vi "Update_Enum (SubVI).vi"(8 "error in":errorcluster, 11 "AppContext in":T1={"VIRefToProcessTemplate"=refnum, "VIRefToThisVI"=refnum, "ProcessesList"=[], "VIRefToEnumProcess"=refnum, "VIRefTogetProcessViPath"=refnum, "ProcessManagement"={"EnumProcessState"=enum."Create process", "ProcessName"="", "PathToProcess"=path ""}, "VIRefToSetup"=refnum, "VIRefToStartProcess"=refnum, "ProcessConfig"={"File Path Control"=path "", "Timeout"=0.0, "viInitString"="", "State"=enum."Closed"}}) -> (0 "error out":errorcluster, 3 "AppContext out":T1={"VIRefToProcessTemplate"=refnum, "VIRefToThisVI"=refnum, "ProcessesList"=[], "VIRefToEnumProcess"=refnum, "VIRefTogetProcessViPath"=refnum, "ProcessManagement"={"EnumProcessState"=enum."Create process", "ProcessName"="", "PathToProcess"=path ""}, "VIRefToSetup"=refnum, "VIRefToStartProcess"=refnum, "ProcessConfig"={"File Path Control"=path "", "Timeout"=0.0, "viInitString"="", "State"=enum."Closed"}})   [LabVIEW 2013]
uses:
  Ctl/AppContext.ctl
  Ctl/EnumProcessState.ctl
  050 - CONFIG/20 - ExternalProcesses/paramsExternalProcesses.ctl
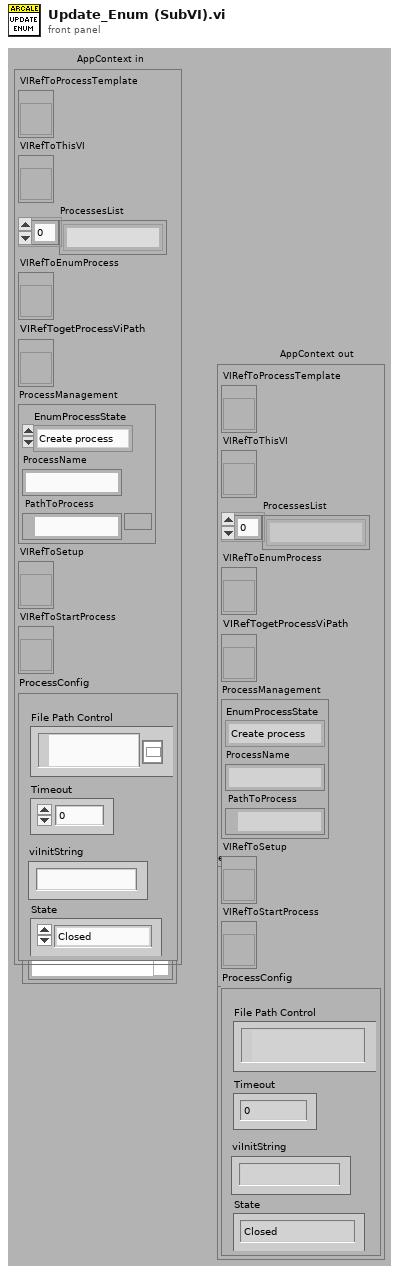
[diagram p1: front panel]
types:
  T1 = typedef "AppContext.ctl" = cluster{"VIRefToProcessTemplate":refnum<vi>, "VIRefToThisVI":refnum<vi>, "ProcessesList":string[], "VIRefToEnumProcess":refnum<vi>, "VIRefTogetProcessViPath":refnum<vi>, "ProcessManagement":cluster{"EnumProcessState":T2, "ProcessName":string, "PathToProcess":path}, "VIRefToSetup":refnum<vi>, "VIRefToStartProcess":refnum<vi>, "ProcessConfig":T3}
  T2 = typedef "EnumProcessState.ctl" = enum16{"Create process", "Delete process"}
  T3 = typedef "paramsExternalProcesses.ctl" = cluster{"File Path Control":path, "Timeout":dbl, "viInitString":string, "State":enum32{"Invalid", "Standard", "Closed", "Hidden", "Minimized", "Maximized"}}
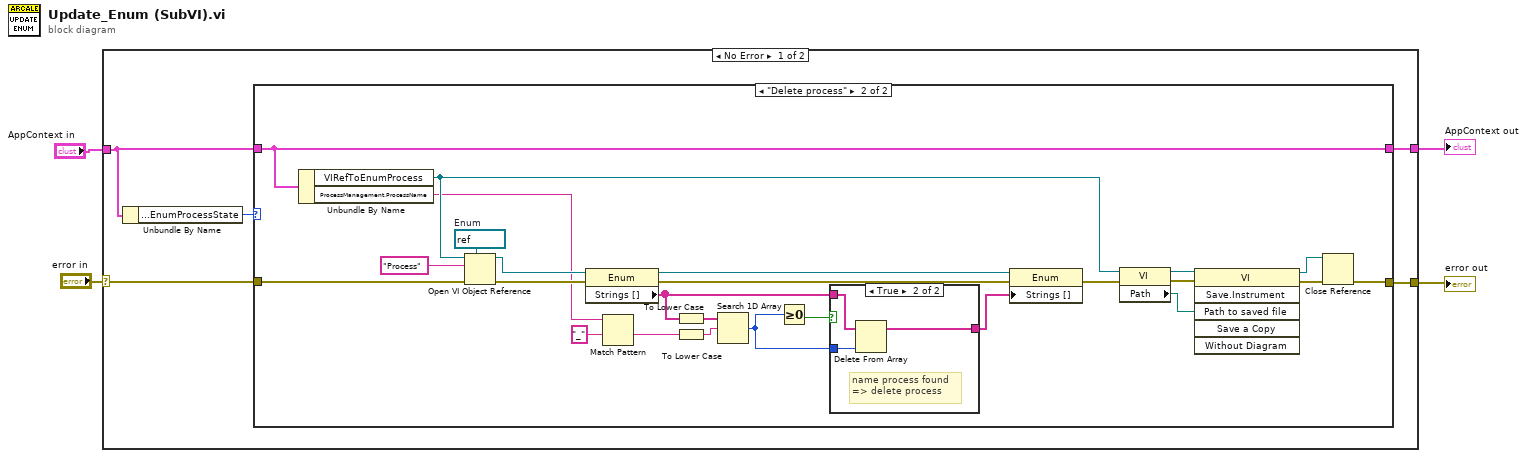
[diagram p0: block diagram]
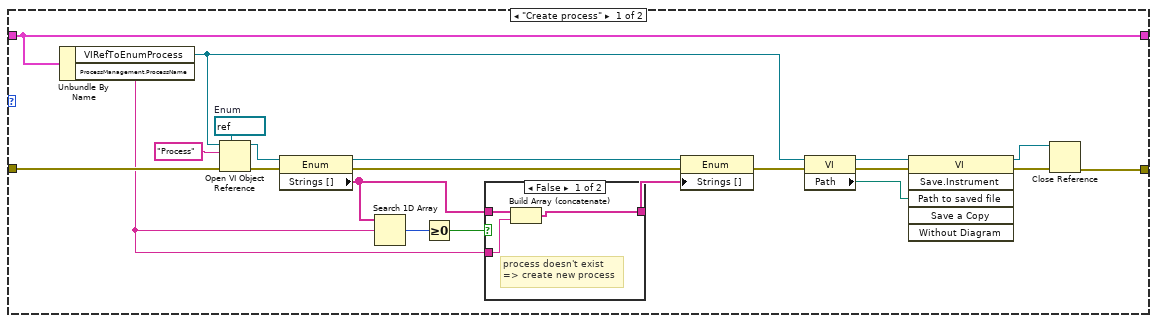
[diagram p2: hidden frame]
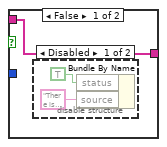
[diagram p4: hidden frame]
diagram:
  n1 = case shown="No Error" "error in" {
    selector: "error in" -> [w5 w66]
    tunnel: [w9 w66] -> w4
    tunnel: "AppContext in" -> [w7 w67]
    tunnel: [w6 w67] -> w2
    frame No Error {
      n2 = Unbundle By Name(w7) -> ("ProcessManagement.EnumProcessState"=w8:T2)
      n3 = case shown="\"Delete process\"" w8 {
        tunnel: w7 -> [w22 w51]
        tunnel: w5 -> [w29 w52]
        tunnel: [w20 w36] -> w9
        tunnel: [w22 w51] -> w6
        frame "Create process" {
          w26 = refnum<vi> refnum  # Enum
          n4 = Unbundle By Name(w22) -> ("VIRefToEnumProcess"=w24:refnum<vi>, "ProcessManagement.ProcessName"=w15:string)
          n5 = Open VI Object Reference(7:w26, 8:w29, 10:"Process" ("name/order"), 11:w24) -> (0:w19:errorcluster, 3:w25:refnum<vi>)
          n6 = property class="Enum"(reference=w25, error in=w19) -> (reference out=w28:refnum<vi>, error out=w27:errorcluster, "Strings []"=w16:string[])
          n7 = Search 1D Array(1D array=w16, element=w15) -> (index of element=w18:i32)  [unwired: 1 in]
          n8 = Greater Or Equal To 0?(x=w18) -> (x >= 0?=w17:bool)
          n9 = case shown="False" w17 {
            tunnel: w16 -> [w33 w34]
            tunnel: w15 -> [w32 _]
            tunnel: [w31 w34] -> w14
            frame False {
              # "process doesn't exist\n=> create new process"
              n10 = Build Array (concatenate)(w33, w32) -> (w31:string[])
            }
            frame True {
            }
          }
          n11 = property class="Enum"(reference=w28, error in=w27, "Strings []"=w14) -> (error out=w12:errorcluster)  [unwired: 1 out]
          n12 = property class="VI"(reference=w24, error in=w12) -> (reference out=w13:refnum<vi>, error out=w11:errorcluster, "Path"=w23:path)
          n13 = invoke class="VI" method="Save.Instrument"(reference=w13, error in=w11, "Path to saved file"=w23) -> (reference out=w21:refnum<vi>, error out=w10:errorcluster)  [unwired: 3 in, 4 out]
          n14 = Close Reference(reference=w21, error in (no error)=w10) -> (error out=w20:errorcluster)
        }
        frame "Delete process" {
          w56 = refnum<vi> refnum  # Enum
          n15 = Unbundle By Name(w51) -> ("VIRefToEnumProcess"=w54:refnum<vi>, "ProcessManagement.ProcessName"=w46:string)
          n16 = Open VI Object Reference(7:w56, 8:w52, 10:"Process" ("name/order"), 11:w54) -> (0:w47:errorcluster, 3:w55:refnum<vi>)
          n17 = property class="Enum"(reference=w55, error in=w47) -> (reference out=w58:refnum<vi>, error out=w57:errorcluster, "Strings []"=w45:string[])
          n18 = Match Pattern(string=w46, regular expression="_") -> (after substring=w44:string)  [unwired: 1 in, 3 out]
          n19 = To Lower Case(string=w45) -> (all lower case string=w49:string[])
          n20 = To Lower Case(string=w44) -> (all lower case string=w43:string)
          n21 = Search 1D Array(1D array=w49, element=w43) -> (index of element=w42:i32)  [unwired: 1 in]
          n22 = Greater Or Equal To 0?(x=w42) -> (x >= 0?=w41:bool)
          n23 = case shown="True" w41 {
            tunnel: w45 -> [w60 w65]
            tunnel: w42 -> [_ w64]
            tunnel: [w60 w63] -> w48
            frame False {
              n24 = disable-structure shown="Disabled" {
                frame Disabled {
                  n25 = Bundle By Name("status"=TRUE, "source"="There is no process with that name.") -> ()  [unwired: 1 in, 1 out]
                }
                frame Enabled {
                }
              }
            }
            frame True {
              # "name process found\n=> delete process"
              n26 = Delete From Array(array=w65, index=w64) -> (array with subset deleted=w63:string[])  [unwired: 1 in, 1 out]
            }
          }
          n27 = property class="Enum"(reference=w58, error in=w57, "Strings []"=w48) -> (error out=w40:errorcluster)  [unwired: 1 out]
          n28 = property class="VI"(reference=w54, error in=w40) -> (reference out=w38:refnum<vi>, error out=w39:errorcluster, "Path"=w53:path)
          n29 = invoke class="VI" method="Save.Instrument"(reference=w38, error in=w39, "Path to saved file"=w53) -> (reference out=w35:refnum<vi>, error out=w37:errorcluster)  [unwired: 3 in, 4 out]
          n30 = Close Reference(reference=w35, error in (no error)=w37) -> (error out=w36:errorcluster)
        }
      }
    }
    frame Error {
    }
  }
  "error out" <- w4
  "AppContext out" <- w2
